vi "Pre Launch Init.vi"(11 "Analog Output Channel in":refnum<class "Analog Output Channel.lvclass">) -> (0 "error out":errorcluster, 3 "Analog Output Channel out":refnum<class "Analog Output Channel.lvclass">)   [LabVIEW 2015, in "Analog Output Channel.lvlib" / "Analog Output Channel.lvclass"]
doc: "(<B>Filename</B>: Actor Framework.lvlib:Actor.lvclass:Pre Launch Init.vi)\n\nDefines behavior that occurs after the Launch Actor method is invoked but before the actor's Actor Core method begins running.\n\nThe Pre Launch Init method is guaranteed to finish before the Launch Actor method returns to its caller and before the actor itself receives any messages. Any references that the Pre Launch Init method obtains are guaranteed to have the same lifetime as the actor itself. Any errors that the Pre Launch Init method returns will abort the launch.\n\nBy default, this method does nothing. A descendant class may override it to define behavior."
uses:
  Analog Output Channel.lvclass
  AOChData.lvclass
  Channel/ChannelData.lvclass
  Output Channel/Output Channel/Output Channel.lvclass
  Channel/Channel/Channel.lvclass
  <vilib>/measure/NI_MABase.lvlib
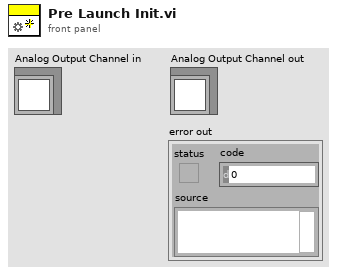
[diagram p1: front panel]
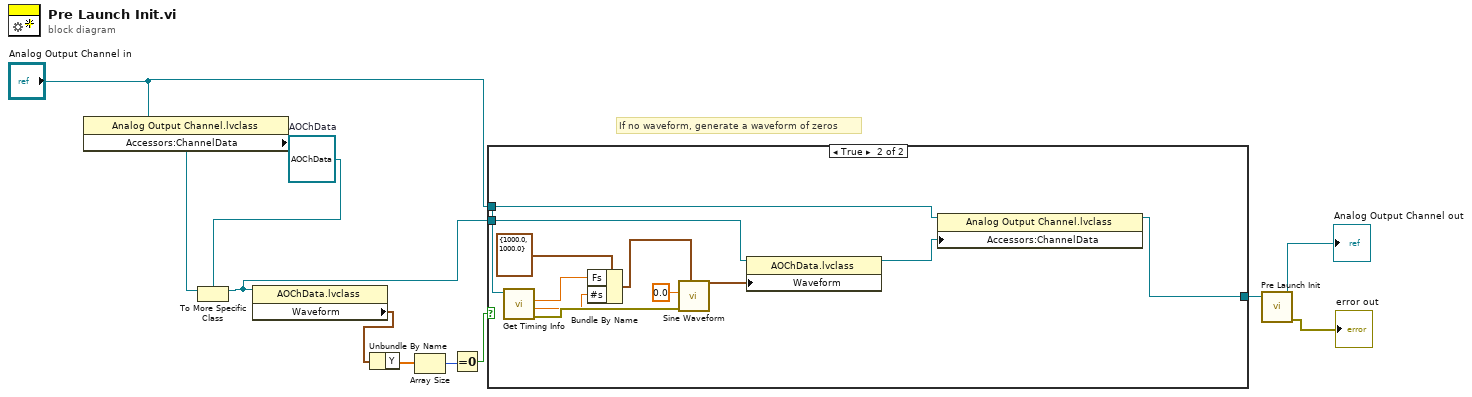
[diagram p0: block diagram]
diagram:
  w9 = refnum<class "AOChData.lvclass"> refnum  # AOChData
  # "If no waveform, generate a waveform of zeros"
  n1 = property class="Analog Output Channel.lvclass"(reference="Analog Output Channel in") -> ("Accessors:ChannelData"=w8:refnum<class "ChannelData.lvclass">)  [unwired: 1 in, 2 out]
  n2 = To More Specific Class(target class=w9, reference=w8) -> (specific class reference=w6:refnum<class "AOChData.lvclass">)  [unwired: 1 in, 1 out]
  n3 = property class="AOChData.lvclass"(reference=w6) -> ("Waveform"=w3:waveform(dbl))  [unwired: 1 in, 2 out]
  n4 = Unbundle By Name(w3) -> ("Y"=w4:dbl[])
  n5 = Array Size(array=w4) -> (size(s)=w2:i32)
  n6 = Equal To 0?(x=w2) -> (x = 0?=w1:bool)
  n7 = case shown="True" w1 {
    tunnel: "Analog Output Channel in" -> [w12 w15]
    tunnel: w6 -> [_ w17]
    tunnel: [w12 w13] -> w5
    frame False {
    }
    frame True {
      n8 = call "Get Timing Info.vi"("Channel in"=w15) -> ("error out"=w23:errorcluster, "Buffer Size"=w19:dbl, "Sample Rate"=w20:dbl)  [unwired: 7 in, 1 out]
      n9 = Bundle By Name(cluster=cluster{"Fs":dbl, "#s":dbl} {"Fs"=1000.0, "#s"=1000.0} ("sampling info"), "Fs"=w20, "#s"=w19) -> (w21:cluster{"Fs":dbl, "#s":dbl})
      n10 = call <vilib>:"Sine Waveform.vi"("sampling info"=w21, "error in (no error)"=w23, "amplitude"=0.0) -> ("signal out"=w16:waveform(dbl))  [unwired: 7 in, 1 out]
      n11 = property class="AOChData.lvclass"(reference=w17, "Waveform"=w16) -> (reference out=w14:refnum<class "AOChData.lvclass">)  [unwired: 1 in, 1 out]
      n12 = property class="Analog Output Channel.lvclass"(reference=w15, "Accessors:ChannelData"=w14) -> (reference out=w13:refnum<class "Analog Output Channel.lvclass">)  [unwired: 1 in, 1 out]
    }
  }
  n13 = call-parent "Pre Launch Init.vi"("Channel in"=w5) -> ("error out"=→"error out":errorcluster, "Channel out"=→"Analog Output Channel out":refnum<class "Analog Output Channel.lvclass">)  [unwired: 9 in]
